vi "LeastDistanceAngle.vi"(2 "current angle (no limits)":dbl, 3 "target angle (between pi and -pi)":dbl(knob) scale=3.14159..-3.14159) -> (0 "Reverse?":bool, 1 "motor output angle":dbl)   [LabVIEW 2014]
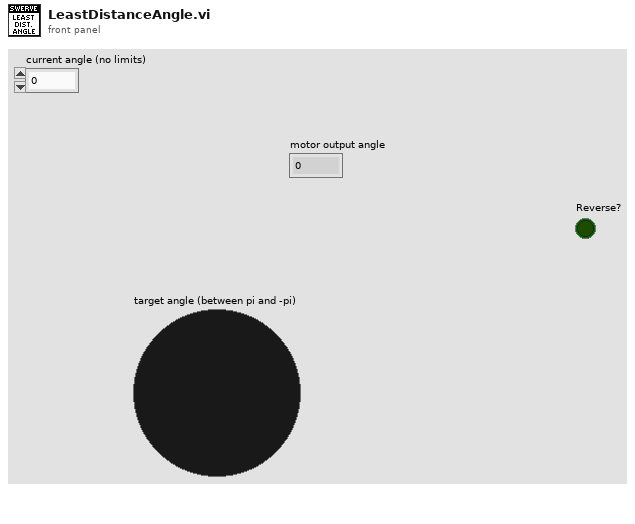
[diagram p1: front panel]
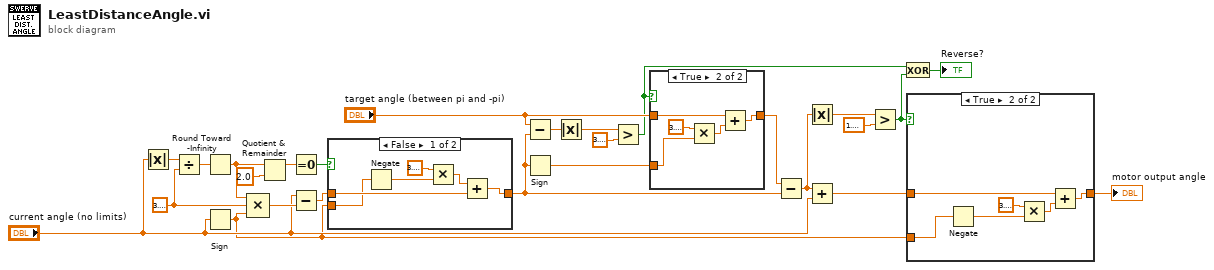
[diagram p0: block diagram]
diagram:
  w23 = 3.141592653589793
  n1 = Absolute Value(x="current angle (no limits)") -> (abs(x)=w26:dbl)
  n2 = Divide(x=w26, y=w23) -> (x/y=w25:dbl)
  n3 = Round Toward -Infinity(1:w25) -> (0:w22:dbl)
  n4 = Sign(1:"current angle (no limits)") -> (0:w11:dbl)
  n5 = Compound Arithmetic op=MULTIPLY(w22, w23, w11) -> (w24:dbl)
  n6 = Quotient & Remainder(x=w22, y=2.0) -> (x-y*floor(x/y)=w20:dbl)  [unwired: 1 out]
  n7 = Equal To 0?(x=w20) -> (x = 0?=w18:bool)
  n8 = Subtract(x="current angle (no limits)", y=w24) -> (x-y=w19:dbl)
  n9 = case shown="False" w18 {
    tunnel: [w31 w33] -> w5
    tunnel: w19 -> [w32 w33]
    tunnel: w11 -> [w30 _]
    frame False {
      n10 = Negate(x=w30) -> (-x=w28:dbl)
      n11 = Multiply(x=3.141592653589793, y=w28) -> (x*y=w27:dbl)
      n12 = Add(x=w27, y=w32) -> (x+y=w31:dbl)
    }
    frame True {
    }
  }
  n13 = Subtract(x="target angle (between pi and -pi)", y=w5) -> (x-y=w14:dbl)
  n14 = Sign(1:w5) -> (0:w4:dbl)
  n15 = Absolute Value(x=w14) -> (abs(x)=w10:dbl)
  n16 = Greater?(x=w10, y=3.141592653589793) -> (0:w2:bool)
  n17 = case shown="True" w2 {
    tunnel: "target angle (between pi and -pi)" -> [w34 w38]
    tunnel: [w34 w39] -> w8
    tunnel: w4 -> [_ w35]
    frame False {
    }
    frame True {
      n18 = Multiply(x=3.141592653589793, y=w35) -> (x*y=w36:dbl)
      n19 = Add(x=w38, y=w36) -> (x+y=w39:dbl)
    }
  }
  n20 = Subtract(x=w8, y=w5) -> (x-y=w7:dbl)
  n21 = Absolute Value(x=w7) -> (abs(x)=w9:dbl)
  n22 = Add(x=w7, y="current angle (no limits)") -> (x+y=w12:dbl)
  n23 = Greater?(x=w9, y=1.5707963267948966) -> (0:w15:bool)
  n24 = Exclusive Or(1:w15, 2:w2) -> (0:→"Reverse?":bool)
  n25 = case shown="True" w15 {
    tunnel: [w40 w46] -> w1
    tunnel: w12 -> [w40 w45]
    tunnel: w11 -> [_ w44]
    frame False {
    }
    frame True {
      n26 = Negate(x=w44) -> (-x=w43:dbl)
      n27 = Multiply(x=3.141592653589793, y=w43) -> (x*y=w41:dbl)
      n28 = Add(x=w45, y=w41) -> (x+y=w46:dbl)
    }
  }
  "motor output angle" <- w1
